vi "WebSocket_Create.vi"(8 "error in (no error)":errorcluster, 10 "Socket":refnum<k5>, 11 "reference in":refnum<class "WebSocket.lvclass">) -> (0 "error out":errorcluster, 3 "reference out":refnum<class "WebSocket.lvclass">)   [LabVIEW 2023, in "WebSocket.lvclass"]
uses:
  WebSocket.lvclass
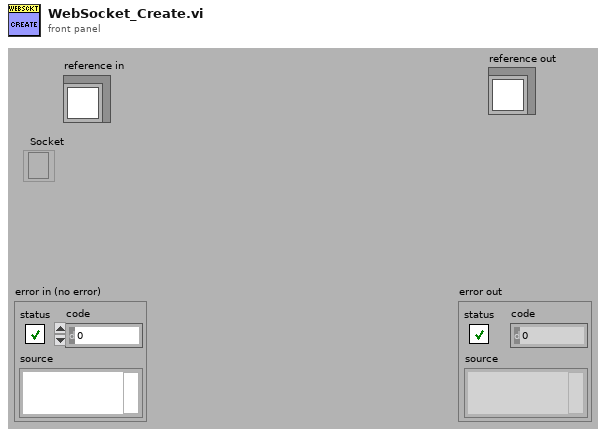
[diagram p1: front panel]
types:
  T1 = typedef "WebSocket.lvclass/ObjectAttributes.ctl" = cluster{"Socket":refnum<k5>, "Thread":refnum<vi>, "From Socket":refnum<queue>, "To Socket":refnum<queue>, "Rx Stats in Progress":variant, "Rx Stats":variant, "Tx Stats in Progress":variant, "Tx Stats":variant}
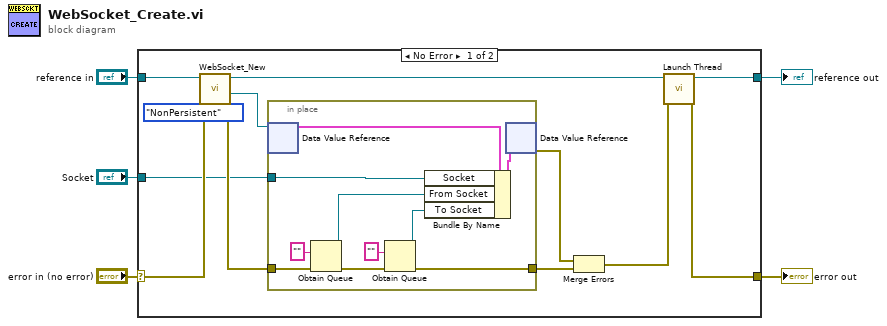
[diagram p0: block diagram]
diagram:
  n1 = case shown="No Error" "error in (no error)" {
    selector: "error in (no error)" -> [w16 w29]
    tunnel: [w7 w29] -> w4
    tunnel: "reference in" -> [w17 w28]
    tunnel: [w6 w28] -> w2
    tunnel: "Socket" -> [w12 _]
    frame No Error {
      n2 = call "WebSocket_New.vi"("Persistent/Debugging(Default)"=enum16{"Default", "Persistent", "NonPersistent"}."NonPersistent", "error in (no error)"=w16, "reference in"=w17) -> ("error out"=w15:errorcluster, "DVRRefOut"=w10:refnum<data-value>, "reference out"=w9:refnum<class "WebSocket.lvclass">)  [unwired: 5 in, 1 out]
      n3 = in-place {
        in-place-border: w15 -> [w23]
        in-place-border: [w18] -> w14
        in-place-border: w12 -> [w25]
        n4 = in-place-dvr #1(w10) -> (w26:T1)  [unwired: 1 out]
        n5 = Obtain Queue(element data type="", error in (no error)=w23) -> (queue out=w21:refnum<queue>, error out=w19:errorcluster)  [unwired: 3 in, 1 out]
        n6 = Obtain Queue(element data type="", error in (no error)=w19) -> (queue out=w20:refnum<queue>, error out=w18:errorcluster)  [unwired: 3 in, 1 out]
        n7 = Bundle By Name(cluster=w26, "Socket"=w25, "From Socket"=w21, "To Socket"=w20) -> (w27:T1)
        n8 = in-place-dvr #1(w27) -> (w11:errorcluster)  [unwired: 1 out]
      }
      n9 = Merge Errors(w11, w14) -> (w8:errorcluster)
      n10 = call-dynamic "Launch Thread.vi"("error in (no error)"=w8, "WebSocket in"=w9) -> ("error out"=w7:errorcluster, "WebSocket out"=w6:refnum<class "WebSocket.lvclass">)  [unwired: 8 in]
    }
    frame Error {
    }
  }
  "error out" <- w4
  "reference out" <- w2
